vi "exp_base.vi"(11 "count":i32) -> (2 "counter":i32)   [LabVIEW 2024]
uses:
  the_counter_fsm37.dll
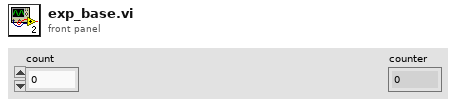
[diagram p1: front panel]
types:
  T1 = enum32{"Bad", "Idle", "Run top level", "Running"}
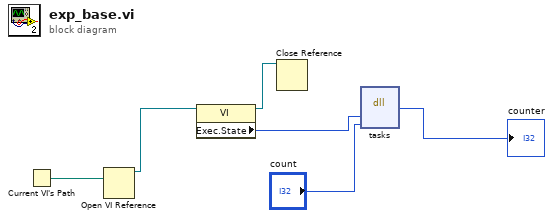
[diagram p0: block diagram]
diagram:
  n1 = Current VI's Path() -> (path=w5:path)
  n2 = Open VI Reference(vi path=w5) -> (vi reference=w2:refnum<vi>)  [unwired: 5 in, 1 out]
  n3 = property class="VI"(reference=w2) -> (reference out=w3:refnum<vi>, "Exec.State"=w1:T1)  [unwired: 1 in, 1 out]
  n4 = Close Reference(reference=w3) -> ()  [unwired: 1 in, 1 out]
  n5 = dll-call lib="D:/nilrt/counter/the_counter_fsm37.dll" fn="tasks"("sig"=w1, "count"="count") -> ("counter"=→"counter":i32)  [unwired: 5 in, 2 out]
